vi "Thread Loop.vi"(8 "error in (no error)":errorcluster, 11 "Car Wash Controller in":refnum<class "Car Wash Controller.lvclass">) -> (0 "error out":errorcluster, 3 "Car Wash Controller out":refnum<class "Car Wash Controller.lvclass">)   [LabVIEW 2012, in "Car Wash Controller.lvlib" / "Car Wash Controller.lvclass"]
uses:
  Car Wash Controller.lvclass
  Thread/Thread.lvclass
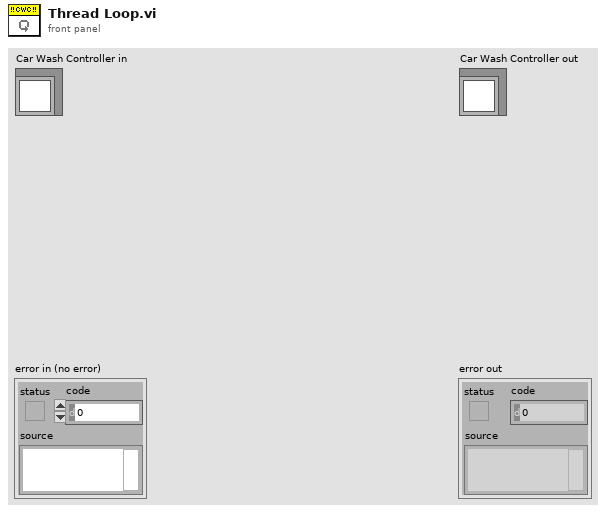
[diagram p1: front panel]
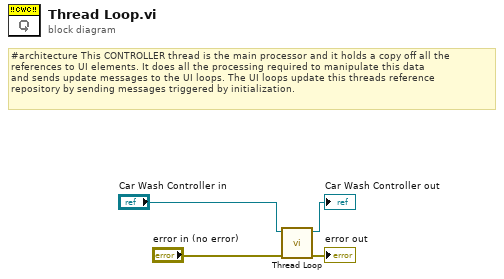
[diagram p0: block diagram]
diagram:
  # "#architecture This CONTROLLER thread is the main processor and it holds a copy off all the \nreferences to UI elements. It does all the processing required to manipulate this data\nand sends update messages to the UI loops. The UI loops update this threads reference\nrepository by sending messages triggered by initialization."
  n1 = call-parent "Thread Loop.vi"("error in (no error)"="error in (no error)", "Thread in"="Car Wash Controller in") -> ("error out"=→"error out":errorcluster, "Thread out"=→"Car Wash Controller out":refnum<class "Car Wash Controller.lvclass">)  [unwired: 8 in]
